vi "re_msg.send_lua.vi"(5 "LuaVIEW reference":T1) -> (15 "error out":errorcluster)   [LabVIEW 2012]
doc: "Sends a message to a task specified via its identifier. This adds the message to the task's message queue and wakes it up if asleep. Since the message is queued, it is possible for multiple messages to be sent without loss when the receiving task is otherwise preoccupied.\nParameters:\nstr:task, identifier of the receiving task.\nstr:message, use a message that the receiving task understands.\nErrors:\nReceiving task does not exist.\nReceiving task is in an error state."
uses:
  typedefs/t_LuaVIEW Reference.ctl
  typedefs/t_LuaVIEW Task List Methods.ctl
  subvis/private/LuaVIEW Pull (string).vi
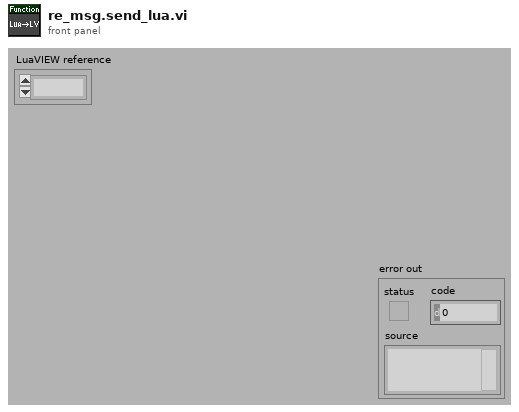
[diagram p1: front panel]
types:
  T1 = typedef "t_LuaVIEW Reference.ctl" = refnum<k1>
  T2 = typedef "t_LuaVIEW Task List Methods.ctl" = enum16{"clear list", "add", "test", "remove", "get ref", "get task info", "get list", "get script info", "ongoing?", "resume", "pause", "stop", "confirm", "message"}
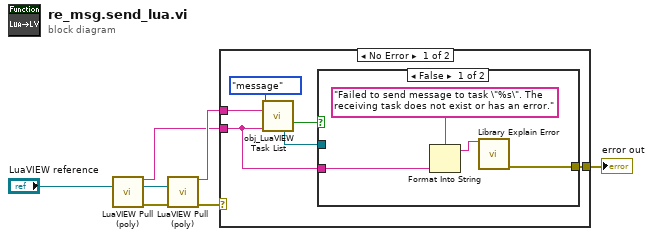
[diagram p0: block diagram]
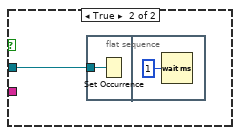
[diagram p2: hidden frame]
diagram:
  n1 = call-poly "LuaVIEW Pull (poly).vi"("LuaVIEW reference in"="LuaVIEW reference") -> ("string"=w3:string, "LuaVIEW reference out"=w5:T1, "error out"=w2:errorcluster)  [unwired: 12 in]
  n2 = call-poly "LuaVIEW Pull (poly).vi"("LuaVIEW reference in"=w5, "error in (no error)"=w2) -> ("string"=w4:string, "error out"=w1:errorcluster)  [unwired: 11 in, 1 out]
  n3 = case shown="No Error" w1 {
    selector: w1 -> [_ w21]
    tunnel: [w13 w21] -> w7
    tunnel: w4 -> [w9 _]
    tunnel: w3 -> [w8 _]
    frame No Error {
      n4 = call "obj_LuaVIEW Task List.vi"("method"=t_LuaVIEW_Task_List_Methods."message", "message"=w9, "task identifier"=w8) -> ("set/ongoing"=w11:bool, "wakeup occurrence"=w10:refnum<k4>)  [unwired: 7 in, 4 out]
      n5 = case shown="False" w11 {
        tunnel: [w15 _] -> w13
        tunnel: w8 -> [w14 _]
        tunnel: w10 -> [_ w18]
        frame False {
          n6 = Format Into String(format string="Failed to send message to task \"%s\". The receiving task does not exist or has an error.", w14) -> (resulting string=w17:string)  [unwired: 2 in, 1 out]
          n7 = call "Library Explain Error.vi"("explanation prefix (none)"=w17) -> ("explained error"=w15:errorcluster)  [unwired: 14 in]
        }
        frame True {
          n8 = flat-sequence {
            tunnel: w18 -> [w19]
            frame #0 {
              n9 = Set Occurrence(w19) -> ()
            }
            frame #1 {
              n10 = Wait (ms)(milliseconds to wait=u32 1) -> ()  [unwired: 1 out]
            }
          }
        }
      }
    }
    frame Error {
    }
  }
  "error out" <- w7
